vi "map.vi"(0 "inmax":dbl=1.0, 5 "inmin":dbl, 7 "outmax":dbl=1.0, 9 "outmin":dbl, 11 "in":dbl[](array[numeric])) -> (15 "out":dbl[](array[numeric]))   [LabVIEW 2019]
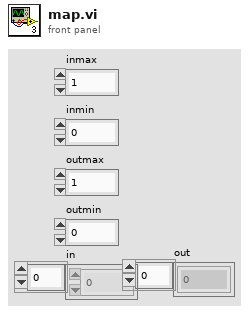
[diagram p1: front panel]
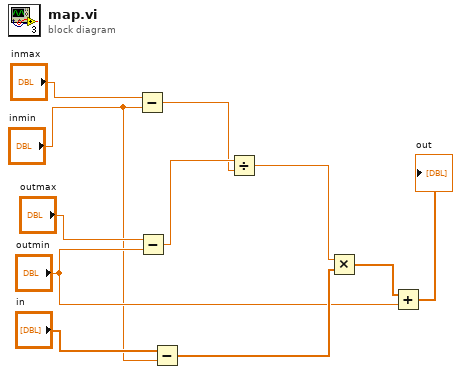
[diagram p0: block diagram]
diagram:
  n1 = Subtract(x="inmax", y="inmin") -> (x-y=w9:dbl)
  n2 = Subtract(x="outmax", y="outmin") -> (x-y=w10:dbl)
  n3 = Subtract(x="in", y="inmin") -> (x-y=w5:dbl[])
  n4 = Divide(x=w10, y=w9) -> (x/y=w6:dbl)
  n5 = Multiply(x=w6, y=w5) -> (x*y=w4:dbl[])
  n6 = Add(x=w4, y="outmin") -> (x+y=→"out":dbl[])
